vi "Corridor Width.vi"(9 "Trial Fraction IN":dbl(slide) scale=0.0..1.0, 10 "Corridor Width Values (mm)":string, 11 "Corridor Width Change Positions":string) -> (3 "Corridor Width (mm)":dbl)   [LabVIEW 2018]
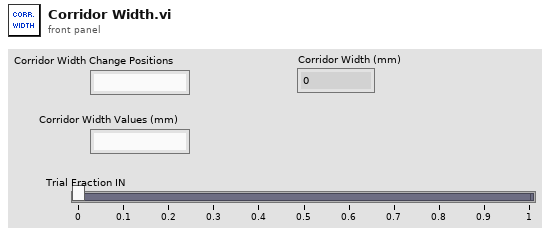
[diagram p1: front panel]
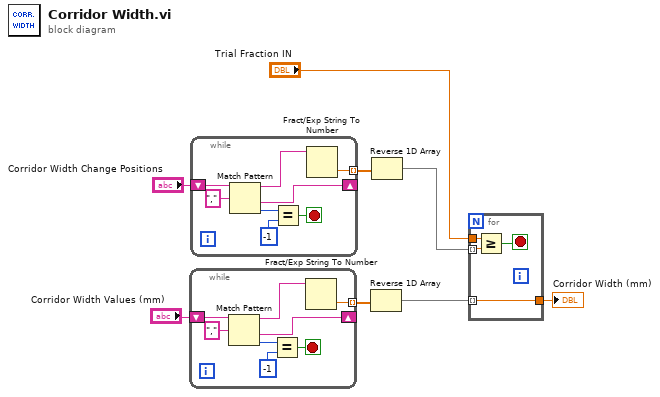
[diagram p0: block diagram]
diagram:
  n1 = while {
    shift-right: [w9] -> _
    shift-left: "Corridor Width Values (mm)" -> [w15]
    tunnel: [w10] -> w3 mode=indexing
    stop <- w12 stop-if-true
    n2 = Match Pattern(string=w15, regular expression=",") -> (before substring=w11:string, after substring=w9:string, offset past match=w14:i32)  [unwired: 1 in, 1 out]
    n3 = Equal?(x=w14, y=-1) -> (x = y?=w12:bool)
    n4 = Fract/Exp String To Number(string=w11) -> (number=w10:dbl)  [unwired: 3 in, 1 out]
  }
  n5 = while {
    shift-right: [w17] -> _
    shift-left: "Corridor Width Change Positions" -> [w23]
    tunnel: [w18] -> w2 mode=indexing
    stop <- w20 stop-if-true
    n6 = Match Pattern(string=w23, regular expression=",") -> (before substring=w19:string, after substring=w17:string, offset past match=w22:i32)  [unwired: 1 in, 1 out]
    n7 = Equal?(x=w22, y=-1) -> (x = y?=w20:bool)
    n8 = Fract/Exp String To Number(string=w19) -> (number=w18:dbl)  [unwired: 3 in, 1 out]
  }
  n9 = Reverse 1D Array(array=w3) -> (reversed array=w7:dbl[])
  n10 = Reverse 1D Array(array=w2) -> (reversed array=w5:dbl[])
  n11 = for {
    tunnel: w5 -> [w28] mode=indexing
    tunnel: "Trial Fraction IN" -> [w26]
    tunnel: w7 -> [w25] mode=indexing
    tunnel: [w25] -> w8
    stop <- w27 stop-if-true
    n12 = Greater Or Equal?(x=w26, y=w28) -> (x >= y?=w27:bool)
  }
  "Corridor Width (mm)" <- w8
